vi "APS arc2 ca all.vi"(0 "Axis_ID_Array":i32, 1 "Option":i32, 2 "CenterArray":dbl, 3 "Angle":dbl, 4 "TransPara":dbl, 5 "Vs":dbl, 6 "Vm":dbl, 7 "error in (no error)":errorcluster caption="错误输入（无错误）", 8 "Ve":dbl, 9 "Acc":dbl, 10 "Dec":dbl, 11 "SFac":dbl, 12 "Wait":cluster{"h_event":u32, "i32_ret":i32}) -> (14 "Wait out":cluster{"h_event":u32, "i32_ret":i32}, 20 "Axis_ID_Array out":i32, 21 "function return":i32, 22 "CenterArray out":dbl, 24 "TransPara out":dbl, 27 "error out":errorcluster caption="错误输出")   [LabVIEW 2011, in "APS168.lvlib"]
doc: "I32 FNTYPE APS_arc2_ca_all( I32 *Axis_ID_Array, I32 Option, F64 *CenterArray, F64 Angle, F64 *TransPara, F64 Vs, F64 Vm, F64 Ve, F64 Acc,F64 Dec, F64 SFac, ASYNCALL *Wait );"
uses:
  APS168.lvlib
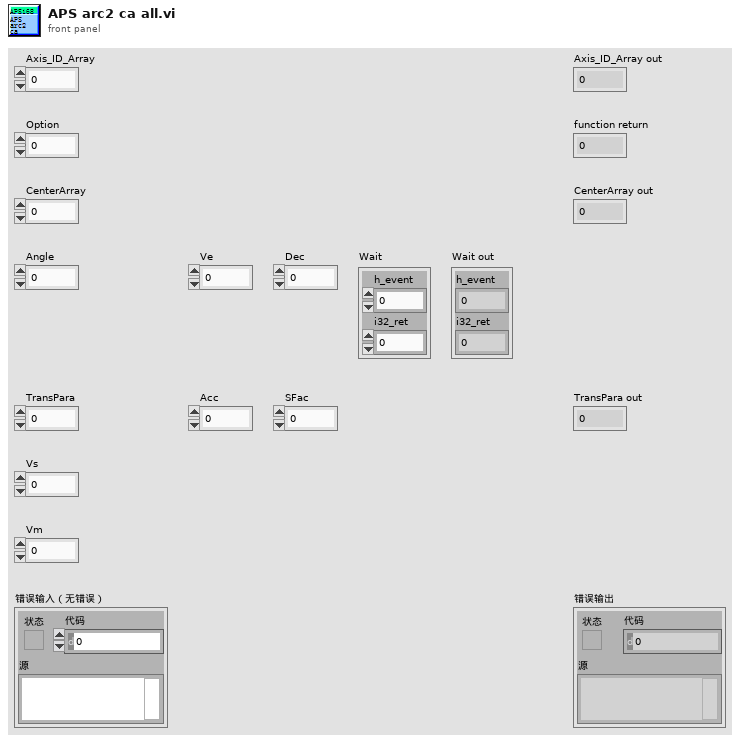
[diagram p1: front panel]
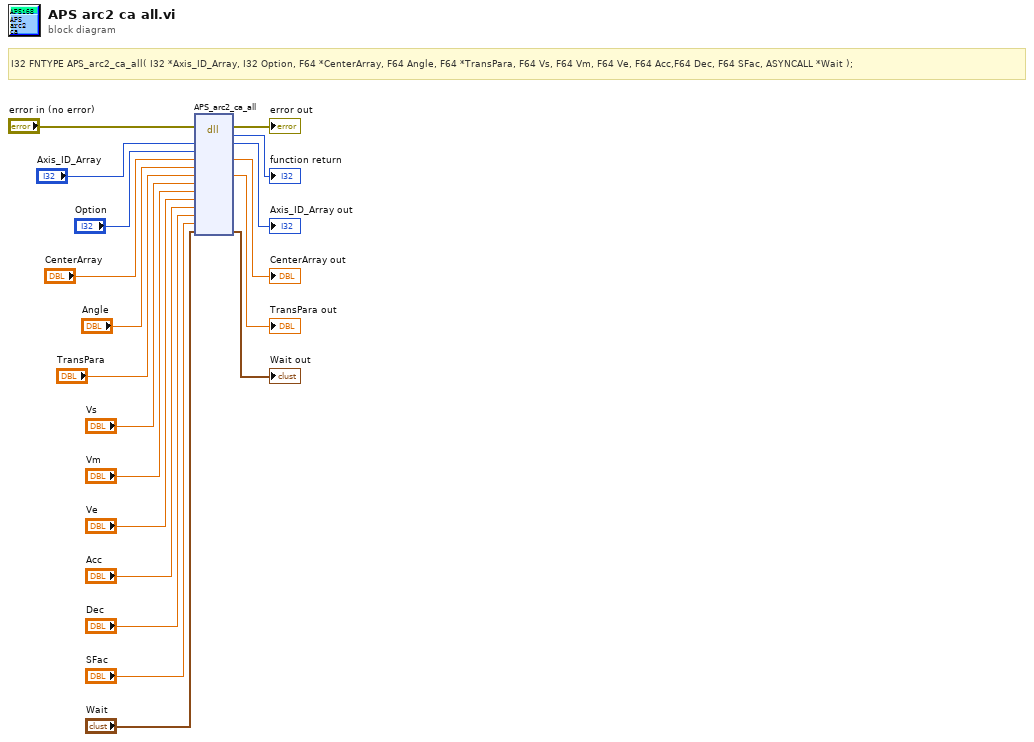
[diagram p0: block diagram]
diagram:
  # "I32 FNTYPE APS_arc2_ca_all( I32 *Axis_ID_Array, I32 Option, F64 *CenterArray, F64 Angle, F64 *TransPara, F64 Vs, F64 Vm, F64 Ve, F64 Acc,F64 Dec, F64 SFac, ASYNCALL *Wait );"
  n1 = dll-call lib="PTH1Labs E软件ADLINK 204CAPS_1_7_1_LIB line 连续运动204APS168.*" fn="APS_arc2_ca_all"(error in="error in (no error)", "Axis_ID_Array"="Axis_ID_Array", "Option"="Option", "CenterArray"="CenterArray", "Angle"="Angle", "TransPara"="TransPara", "Vs"="Vs", "Vm"="Vm", "Ve"="Ve", "Acc"="Acc", "Dec"="Dec", "SFac"="SFac", "Wait"="Wait") -> (error out=→"error out":errorcluster, →"function return":i32, "Axis_ID_Array"=→"Axis_ID_Array out":i32, "CenterArray"=→"CenterArray out":dbl, "TransPara"=→"TransPara out":dbl, "Wait"=→"Wait out":cluster{"h_event":u32, "i32_ret":i32})  [unwired: 10 in, 1 out]
